vi "Read from Config File-Rev4.vi"(4 "error in (no error)":errorcluster, 5 "Measurement Information In":T4={"Comments"="", "Directory Input"="", "Data file path"=path "C:/Data/EPR Data", "Scripting File"=path "C:/Data/Configuration Script.csv", "Save Data"=FALSE, "Tooth size (d11) [mm]"=0.0, "Tooth size (d12) [mm]"=0.0, "Tooth size (d21) [mm]"=0.0, "Tooth size (d22) [mm]"=0.0, "Dose of Tooth [Gy]"=0.0, "Safe Shutdown?"=FALSE, "Gases Available"=[], "Database Username"="", "Database Password"="", "Database Login URL"="", "Database Upload URL"="", "Database Success URL"="", "Database XML URL"="", "Database Resonator URL"="", "Session Number"=0, "Set #"=0, "Resonator Operator"="", "Session Type"="", "Tooth/Sample ID"="", "Volunteer ID"="", "Computer Operator"="", "Volunteer Type"="", "Site/Tooth Selection (T8,T9)"="", "Resonator"="", "Measurement Site"="", "Non-standard session?"=FALSE, "EPR DAQ Version"="", "Session Path"=path "C:/Data/EPR Data", "Chosen Applied State"="", "Chosen Initial State"="", "Time of Transition"="", "DAQ Mode"=enum."Engineering", "pO2/Scan [mmHg]"=[], "pO2/Set [mmHg]"=[], "Linewidth (HWHM)/Scan [Gauss]"=[], "Linewidth (HWHM)/Set [Gauss]"=[], "pO2 Conversion"="", "Dose Calibration Cluster"={"Dose Response"={"grand_mean"=0.0292016, "slope"=0.0188720543}, "Dose Correction"={"Sex"=1, "a0"=7.719669421, "a1"=-2.746550736, "a2"=-0.186490355, "a3"=0.041922063, "a4"=-0.849147359, "a5"=0.14330063, "a6"=0.019930219, "A_n"=40.0, "H_n"=10.12, "Dose Correction"=FALSE}, "Dose Reporting"={"Reporting is"=TRUE, "sd_threshold [AU]"=0.06, "sd_model [Gy]"=0.66, "dosimetric_threshold [Gy]"=2.0, "Add intrasession errors is"=FALSE, "Prior Radiation?"=FALSE}}, "OxyChip Slope"=0.0, "OxyChip Intercept"=0.0, "QA Mode"=enum."Select QA Mode", "QA Session?"=FALSE, "Sample Type"=enum."Empty Resonator", "Report pO2/Scan"=FALSE, "Skip End Session Save"=FALSE, "Number of sites"=enum."# Probes", "Recipient Name"="", "Sender Name"="", "Recipient Email"="", "Transition State History"=[], "pO2 Report Times"=[], "Temperature [C]"=0.0, "+Error pO2/Scan [mmHg]"=[], "-Error pO2/Scan [mmHg]"=[], "+Error pO2/Set [mmHg]"=[], "-Error pO2/Set [mmHg]"=[], "Oxy Phase Exclusion Tolerance [rad]"=0.0, "Oxy Center Exclusion Tolerance [%]"=0.0, "Oxy Exclude Unacceptable"=FALSE, "Oxy Unacceptable Estimate Flags"=[], "Save Session PPT"=FALSE, "Flagged Bad Sets"=[]} {"Oxy Center Exclusion Tolerance [%]" format="%#_9g"; "Oxy Phase Exclusion Tolerance [rad]" format="%#_9g"; "Temperature [C]" format="%#_9g"; "OxyChip Intercept" format="%#_9g"; "OxyChip Slope" format="%#_9g"; "Dose Calibration Cluster"."Dose Reporting"."dosimetric_threshold [Gy]" format="%#_9g"; "Dose Calibration Cluster"."Dose Reporting"."sd_model [Gy]" format="%#_9g"; "Dose Calibration Cluster"."Dose Reporting"."sd_threshold [AU]" format="%#_9g"; "Dose Calibration Cluster"."Dose Correction"."H_n" format="%#_9g"; "Dose Calibration Cluster"."Dose Correction"."A_n" format="%#_9g"; "Dose Calibration Cluster"."Dose Correction"."a6" format="%#.9g"; "Dose Calibration Cluster"."Dose Correction"."a5" format="%#.9g"; "Dose Calibration Cluster"."Dose Correction"."a4" format="%#.9g"; "Dose Calibration Cluster"."Dose Correction"."a3" format="%#.9g"; "Dose Calibration Cluster"."Dose Correction"."a2" format="%#.9g"; "Dose Calibration Cluster"."Dose Correction"."a1" format="%#.9g"; "Dose Calibration Cluster"."Dose Correction"."a0" format="%#.9g"; "Dose Calibration Cluster"."Dose Correction"."Sex" items=["Male"=1, "Female"=0]; "Dose Calibration Cluster"."Dose Response"."slope" format="%#_9g"; "Dose Calibration Cluster"."Dose Response"."grand_mean" format="%#_9g"}, 6 "Hardware Parameters In":T3={"Scan Calibration [G/V]"=0.0, "Modulation Calibration [G/V]"=0.0, "Modulation Phase [deg]"=0.0, "Modulation Frequency [Hz]"=0.0, "Attenuation [dB]"=0, "Input Channel Count"=0, "Time constant"=7, "Sensitivity"=17, "Frequency Output Voltage [V]"=0.0, "Phase Output Voltage [V]"=0.0, "Lock-in Offset Compensation"=FALSE, "RF [GHz]"=0.0, "Q Start"=0.0, "Q End"=0.0, "Balance"=0.0, "Phase Error"=0.0, "AFC Error"=0.0, "AFC"=FALSE, "Magnet Rotation"=FALSE, "Balance Scaling Factor"=1.0, "Phase Error Scaling Factor"=1.0, "AFC Error Scaling Factor"=1.0, "Frequency Counter ID"="", "Sweep Waveform"=enum."Sawtooth", "Q-Factor Scale"=0.0, " Q-Data Scale"=0.0, " Q-Data Offset"=0.0, "Magnet Rotation Slope"=0.0, "Magnet Rotation Offset"=0.0, "Phase Sweep Resolution"=0.0, "Hardware Version Number"="", "Spectrometer ID Number"=0, "Spectrometer Name"="", "Lock in Saturation"=0.0, "Balance Threshold"=0.0, "Phase Error Threshold"=0.0, "AFC Error Threshold"=0.0, "Linear Actuator Length"=0.0, "Lock-in OK?"=FALSE, "Ignore Lock-in Comm. Failure"=FALSE, "Gradient Addresses"=[], "Gradient Calibrations [G/A*mm]"=[], "Gradient Power Supplies"=[], "Lock-in Address"="", "Magnet Type"=enum."RRI", "Camera Names"=[], "Sweep Limit [Gauss]"=0.0, "Modulation Limit [Gauss]"=0.0, "Balance Threshold Exceeded?"=FALSE, "Phase Threshold Exceeded?"=FALSE, "AFC Threshold Exceeded?"=FALSE, "Consecutive Re-tune attempts"=0, "Reverse Sweep Slope [sec]"=0.0, "Reverse Sweep Offset [G]"=0.0, "AFC Field Correction [V/MHz]"=0.0, "Active Gradients (X Y Z)"=[], "SpO2 Calibration [SpO2/V]"=1.0, "Heart Rate Calibration [BPM/V]"=1.0, "Thermocouple Channel"=""} {"Sensitivity" items=["", "2 nV", "5 nV", "10 nV", "20 nV", "50 nV", "100 nV", "200 nV", "500 nV", "1 uV", "2 uV", "5 uV", "10 uV", "20 uV", "50 uV", "100 uV", "200 uV", "500 uV", "1 mV", "2 mV", "5 mV", "10 mV", "20 mV", "50 mV", "100 mV", "200 mV", "500 mV", "1 V"]; "Time constant" items=["10 us", "20 us", "40 us", "80 us", "160 us", "320 us", "640 us", "5 ms", "10 ms", "20 ms", "50 ms", "100 ms", "200 ms", "500 ms", "1 s", "2 s", "5 s", "10 s", "20 s", "50 s", "100 s", "200 s", "500 s", "1 ks", "2 ks", "5 ks", "10 ks", "20 ks", "50 ks", "100 ks"]}, 7 "Acquisition Parameters In":T2={"Magnet Angle [deg]"=0.0, "Magnet Angles [deg]"=[], "DeltaVpp [v]"=0.0, "SEM [v]"=0.0, "DeltaVpp Thresh [v]"=0.0, "SEM Thresh [v]"=0.0, "Adaptive Processing"=FALSE, "Acquire Q"=FALSE, "Acquire Photos"=FALSE, "Adaptive Tuning"=FALSE, "Automated Matching"=FALSE, "X-Gradient [G/mm]"=0.0, "Y-Gradient [G/mm]"=0.0, "Z-Gradient [G/mm]"=0.0, "Central Field [G]"=0.0, "Scan Width [G]"=0.0, "Mod. Amp. [G]"=0.0, "Scan Time [s]"=0.0, "Pre-Scan Delay [ms]"=0, "Measurement Timeout [s]"=0.0, "Electromagnet Main Field [G]"=0.0, "Locked Central Field [G]"=0.0, "Scans Excluded"=0, "Scans Completed"=0, "No. Scans/Set"=0, "No. Scans for SNR"=0, "Field Locked Frequency [GHz]"=0.0, "Auto Set-based Field Center"=FALSE, "Prompt for oxy acquisition updates"=FALSE, "Oxy QA Scan?"=FALSE, "Exclude Bad Data"=FALSE, "Optimizing RF Power"=FALSE, "Gradients on/off"=FALSE, "Running Script"=TRUE, "Opto-Coupler Current [A]"=0.0, "Continuous Sweeping"=FALSE, "Sweep Rise Time [sec]"=0, "Reverse Sweep Central Field [G]"=0.0, "Forward Sweep Central Field [G]"=0.0, "Sweep Calibrated"=FALSE, "Modulation Calibrated"=FALSE, "First CheckCal Scan?"=FALSE, "AFC Field Correction"=FALSE, "OxyQAInit Scan Width [G]"=0.0, "OxyQAInit Mod. Amp. [G]"=0.0, "Scans Completed/Session"=0, "Acquire SpO2"=FALSE, "Acquire Temperature"=FALSE, "Over Mod"=FALSE} {"OxyQAInit Mod. Amp. [G]" min=0.0; "OxyQAInit Scan Width [G]" min=0.0; "Mod. Amp. [G]" min=0.0; "Scan Width [G]" min=0.0; "Central Field [G]" min=0.0; "Measurement Timeout [s]" min=0.0; "Scan Time [s]" min=0.0; "Z-Gradient [G/mm]" min=0.0; "SEM Thresh [v]" min=0.0; "SEM [v]" min=0.0; "DeltaVpp [v]" min=0.0}) -> (0 "error out":errorcluster, 1 "Measurement Information Out":T4={"Comments"="", "Directory Input"="", "Data file path"=path "C:/Data/EPR Data", "Scripting File"=path "C:/Data/Configuration Script.csv", "Save Data"=FALSE, "Tooth size (d11) [mm]"=0.0, "Tooth size (d12) [mm]"=0.0, "Tooth size (d21) [mm]"=0.0, "Tooth size (d22) [mm]"=0.0, "Dose of Tooth [Gy]"=0.0, "Safe Shutdown?"=FALSE, "Gases Available"=[], "Database Username"="", "Database Password"="", "Database Login URL"="", "Database Upload URL"="", "Database Success URL"="", "Database XML URL"="", "Database Resonator URL"="", "Session Number"=0, "Set #"=0, "Resonator Operator"="", "Session Type"="", "Tooth/Sample ID"="", "Volunteer ID"="", "Computer Operator"="", "Volunteer Type"="", "Site/Tooth Selection (T8,T9)"="", "Resonator"="", "Measurement Site"="", "Non-standard session?"=FALSE, "EPR DAQ Version"="", "Session Path"=path "C:/Data/EPR Data", "Chosen Applied State"="", "Chosen Initial State"="", "Time of Transition"="", "DAQ Mode"=enum."Engineering", "pO2/Scan [mmHg]"=[], "pO2/Set [mmHg]"=[], "Linewidth (HWHM)/Scan [Gauss]"=[], "Linewidth (HWHM)/Set [Gauss]"=[], "pO2 Conversion"="", "Dose Calibration Cluster"={"Dose Response"={"grand_mean"=0.0292016, "slope"=0.0188720543}, "Dose Correction"={"Sex"=1, "a0"=7.719669421, "a1"=-2.746550736, "a2"=-0.186490355, "a3"=0.041922063, "a4"=-0.849147359, "a5"=0.14330063, "a6"=0.019930219, "A_n"=40.0, "H_n"=10.12, "Dose Correction"=FALSE}, "Dose Reporting"={"Reporting is"=TRUE, "sd_threshold [AU]"=0.06, "sd_model [Gy]"=0.66, "dosimetric_threshold [Gy]"=2.0, "Add intrasession errors is"=FALSE, "Prior Radiation?"=FALSE}}, "OxyChip Slope"=0.0, "OxyChip Intercept"=0.0, "QA Mode"=enum."Select QA Mode", "QA Session?"=FALSE, "Sample Type"=enum."Empty Resonator", "Report pO2/Scan"=FALSE, "Skip End Session Save"=FALSE, "Number of sites"=enum."# Probes", "Recipient Name"="", "Sender Name"="", "Recipient Email"="", "Transition State History"=[], "pO2 Report Times"=[], "Temperature [C]"=0.0, "+Error pO2/Scan [mmHg]"=[], "-Error pO2/Scan [mmHg]"=[], "+Error pO2/Set [mmHg]"=[], "-Error pO2/Set [mmHg]"=[], "Oxy Phase Exclusion Tolerance [rad]"=0.0, "Oxy Center Exclusion Tolerance [%]"=0.0, "Oxy Exclude Unacceptable"=FALSE, "Oxy Unacceptable Estimate Flags"=[], "Save Session PPT"=FALSE, "Flagged Bad Sets"=[]} {"Oxy Center Exclusion Tolerance [%]" format="%#_9g"; "Oxy Phase Exclusion Tolerance [rad]" format="%#_9g"; "Temperature [C]" format="%#_9g"; "OxyChip Intercept" format="%#_9g"; "OxyChip Slope" format="%#_9g"; "Dose Calibration Cluster"."Dose Reporting"."dosimetric_threshold [Gy]" format="%#_9g"; "Dose Calibration Cluster"."Dose Reporting"."sd_model [Gy]" format="%#_9g"; "Dose Calibration Cluster"."Dose Reporting"."sd_threshold [AU]" format="%#_9g"; "Dose Calibration Cluster"."Dose Correction"."H_n" format="%#_9g"; "Dose Calibration Cluster"."Dose Correction"."A_n" format="%#_9g"; "Dose Calibration Cluster"."Dose Correction"."a6" format="%#.9g"; "Dose Calibration Cluster"."Dose Correction"."a5" format="%#.9g"; "Dose Calibration Cluster"."Dose Correction"."a4" format="%#.9g"; "Dose Calibration Cluster"."Dose Correction"."a3" format="%#.9g"; "Dose Calibration Cluster"."Dose Correction"."a2" format="%#.9g"; "Dose Calibration Cluster"."Dose Correction"."a1" format="%#.9g"; "Dose Calibration Cluster"."Dose Correction"."a0" format="%#.9g"; "Dose Calibration Cluster"."Dose Correction"."Sex" items=["Male"=1, "Female"=0]; "Dose Calibration Cluster"."Dose Response"."slope" format="%#_9g"; "Dose Calibration Cluster"."Dose Response"."grand_mean" format="%#_9g"}, 2 "Hardware Parameters Out":T3={"Scan Calibration [G/V]"=0.0, "Modulation Calibration [G/V]"=0.0, "Modulation Phase [deg]"=0.0, "Modulation Frequency [Hz]"=0.0, "Attenuation [dB]"=0, "Input Channel Count"=0, "Time constant"=7, "Sensitivity"=17, "Frequency Output Voltage [V]"=0.0, "Phase Output Voltage [V]"=0.0, "Lock-in Offset Compensation"=FALSE, "RF [GHz]"=0.0, "Q Start"=0.0, "Q End"=0.0, "Balance"=0.0, "Phase Error"=0.0, "AFC Error"=0.0, "AFC"=FALSE, "Magnet Rotation"=FALSE, "Balance Scaling Factor"=1.0, "Phase Error Scaling Factor"=1.0, "AFC Error Scaling Factor"=1.0, "Frequency Counter ID"="", "Sweep Waveform"=enum."Sawtooth", "Q-Factor Scale"=0.0, " Q-Data Scale"=0.0, " Q-Data Offset"=0.0, "Magnet Rotation Slope"=0.0, "Magnet Rotation Offset"=0.0, "Phase Sweep Resolution"=0.0, "Hardware Version Number"="", "Spectrometer ID Number"=0, "Spectrometer Name"="", "Lock in Saturation"=0.0, "Balance Threshold"=0.0, "Phase Error Threshold"=0.0, "AFC Error Threshold"=0.0, "Linear Actuator Length"=0.0, "Lock-in OK?"=FALSE, "Ignore Lock-in Comm. Failure"=FALSE, "Gradient Addresses"=[], "Gradient Calibrations [G/A*mm]"=[], "Gradient Power Supplies"=[], "Lock-in Address"="", "Magnet Type"=enum."RRI", "Camera Names"=[], "Sweep Limit [Gauss]"=0.0, "Modulation Limit [Gauss]"=0.0, "Balance Threshold Exceeded?"=FALSE, "Phase Threshold Exceeded?"=FALSE, "AFC Threshold Exceeded?"=FALSE, "Consecutive Re-tune attempts"=0, "Reverse Sweep Slope [sec]"=0.0, "Reverse Sweep Offset [G]"=0.0, "AFC Field Correction [V/MHz]"=0.0, "Active Gradients (X Y Z)"=[], "SpO2 Calibration [SpO2/V]"=1.0, "Heart Rate Calibration [BPM/V]"=1.0, "Thermocouple Channel"=""} {"Sensitivity" items=["", "2 nV", "5 nV", "10 nV", "20 nV", "50 nV", "100 nV", "200 nV", "500 nV", "1 uV", "2 uV", "5 uV", "10 uV", "20 uV", "50 uV", "100 uV", "200 uV", "500 uV", "1 mV", "2 mV", "5 mV", "10 mV", "20 mV", "50 mV", "100 mV", "200 mV", "500 mV", "1 V"]; "Time constant" items=["10 us", "20 us", "40 us", "80 us", "160 us", "320 us", "640 us", "5 ms", "10 ms", "20 ms", "50 ms", "100 ms", "200 ms", "500 ms", "1 s", "2 s", "5 s", "10 s", "20 s", "50 s", "100 s", "200 s", "500 s", "1 ks", "2 ks", "5 ks", "10 ks", "20 ks", "50 ks", "100 ks"]}, 3 "Acquisition Parameters Out":T2={"Magnet Angle [deg]"=0.0, "Magnet Angles [deg]"=[], "DeltaVpp [v]"=0.0, "SEM [v]"=0.0, "DeltaVpp Thresh [v]"=0.0, "SEM Thresh [v]"=0.0, "Adaptive Processing"=FALSE, "Acquire Q"=FALSE, "Acquire Photos"=FALSE, "Adaptive Tuning"=FALSE, "Automated Matching"=FALSE, "X-Gradient [G/mm]"=0.0, "Y-Gradient [G/mm]"=0.0, "Z-Gradient [G/mm]"=0.0, "Central Field [G]"=0.0, "Scan Width [G]"=0.0, "Mod. Amp. [G]"=0.0, "Scan Time [s]"=0.0, "Pre-Scan Delay [ms]"=0, "Measurement Timeout [s]"=0.0, "Electromagnet Main Field [G]"=0.0, "Locked Central Field [G]"=0.0, "Scans Excluded"=0, "Scans Completed"=0, "No. Scans/Set"=0, "No. Scans for SNR"=0, "Field Locked Frequency [GHz]"=0.0, "Auto Set-based Field Center"=FALSE, "Prompt for oxy acquisition updates"=FALSE, "Oxy QA Scan?"=FALSE, "Exclude Bad Data"=FALSE, "Optimizing RF Power"=FALSE, "Gradients on/off"=FALSE, "Running Script"=TRUE, "Opto-Coupler Current [A]"=0.0, "Continuous Sweeping"=FALSE, "Sweep Rise Time [sec]"=0, "Reverse Sweep Central Field [G]"=0.0, "Forward Sweep Central Field [G]"=0.0, "Sweep Calibrated"=FALSE, "Modulation Calibrated"=FALSE, "First CheckCal Scan?"=FALSE, "AFC Field Correction"=FALSE, "OxyQAInit Scan Width [G]"=0.0, "OxyQAInit Mod. Amp. [G]"=0.0, "Scans Completed/Session"=0, "Acquire SpO2"=FALSE, "Acquire Temperature"=FALSE, "Over Mod"=FALSE} {"OxyQAInit Mod. Amp. [G]" min=0.0; "OxyQAInit Scan Width [G]" min=0.0; "Mod. Amp. [G]" min=0.0; "Scan Width [G]" min=0.0; "Central Field [G]" min=0.0; "Measurement Timeout [s]" min=0.0; "Scan Time [s]" min=0.0; "Z-Gradient [G/mm]" min=0.0; "SEM Thresh [v]" min=0.0; "SEM [v]" min=0.0; "DeltaVpp [v]" min=0.0})   [LabVIEW 2016]
uses:
  Types/Acquisition Parameters.ctl
  Types/Hardware Parameters.ctl
  Types/Measurement Information.ctl
  Analysis/Dose Calculation and Reporting/Dose Calculation Control.ctl
  Types/Sample Type.ctl
  DAQ Management/Get Key Double.vi
  DAQ Management/Get Key U32.vi
  DAQ Management/Get Key String.vi
  DAQ Management/Get Key Bool.vi
  DAQ Management/Get Key I32.vi
  DAQ Management/Get Key Path.vi
panel:
  in  "Dose Calibration Cluster":T1={"Dose Response"={"grand_mean"=0.0292016, "slope"=0.0188720543}, "Dose Correction"={"Sex"=1, "a0"=7.719669421, "a1"=-2.746550736, "a2"=-0.186490355, "a3"=0.041922063, "a4"=-0.849147359, "a5"=0.14330063, "a6"=0.019930219, "A_n"=40.0, "H_n"=10.12, "Dose Correction"=FALSE}, "Dose Reporting"={"Reporting is"=TRUE, "sd_threshold [AU]"=0.06, "sd_model [Gy]"=0.66, "dosimetric_threshold [Gy]"=2.0, "Add intrasession errors is"=FALSE, "Prior Radiation?"=FALSE}} {"Dose Reporting"."dosimetric_threshold [Gy]" format="%#_9g"; "Dose Reporting"."sd_model [Gy]" format="%#_9g"; "Dose Reporting"."sd_threshold [AU]" format="%#_9g"; "Dose Correction"."H_n" format="%#_9g"; "Dose Correction"."A_n" format="%#_9g"; "Dose Correction"."a6" format="%#.9g"; "Dose Correction"."a5" format="%#.9g"; "Dose Correction"."a4" format="%#.9g"; "Dose Correction"."a3" format="%#.9g"; "Dose Correction"."a2" format="%#.9g"; "Dose Correction"."a1" format="%#.9g"; "Dose Correction"."a0" format="%#.9g"; "Dose Correction"."Sex" items=["Male"=1, "Female"=0]; "Dose Response"."slope" format="%#_9g"; "Dose Response"."grand_mean" format="%#_9g"}
  # "Gradients"
  # "Field"
  # "Scans and Sets"
  # "Timing"
  # "Adaptive Dosimetric \nData Processing"
  # "Bridge I/O"
  # "Magnet Rotation"
  # "Field Calibration"
  # "Lock In Amplifier"
  # "Spectrometer Information"
  # "DAQ Settings"
  # "Gradient Coils and Field"
  # "X"
  # "Y"
  # "Z"
  # "Q-Measurements"
  # "Session Information"
  # "Oximetric Data and Information"
  # "Email"
  # "Tooth Information"
  # "Database"
  # "Session Information"
  # "Oximetric Data and Information"
  # "Email"
  # "Tooth Information"
  # "Database"
  # "Bridge I/O"
  # "Magnet Rotation"
  # "Field Calibration"
  # "Lock In Amplifier"
  # "Spectrometer Information"
  # "DAQ Settings"
  # "Gradient Coils and Field"
  # "X"
  # "Y"
  # "Z"
  # "Q-Measurements"
  # "Gradients"
  # "Field"
  # "Scans and Sets"
  # "Timing"
  # "Adaptive Dosimetric \nData Processing"
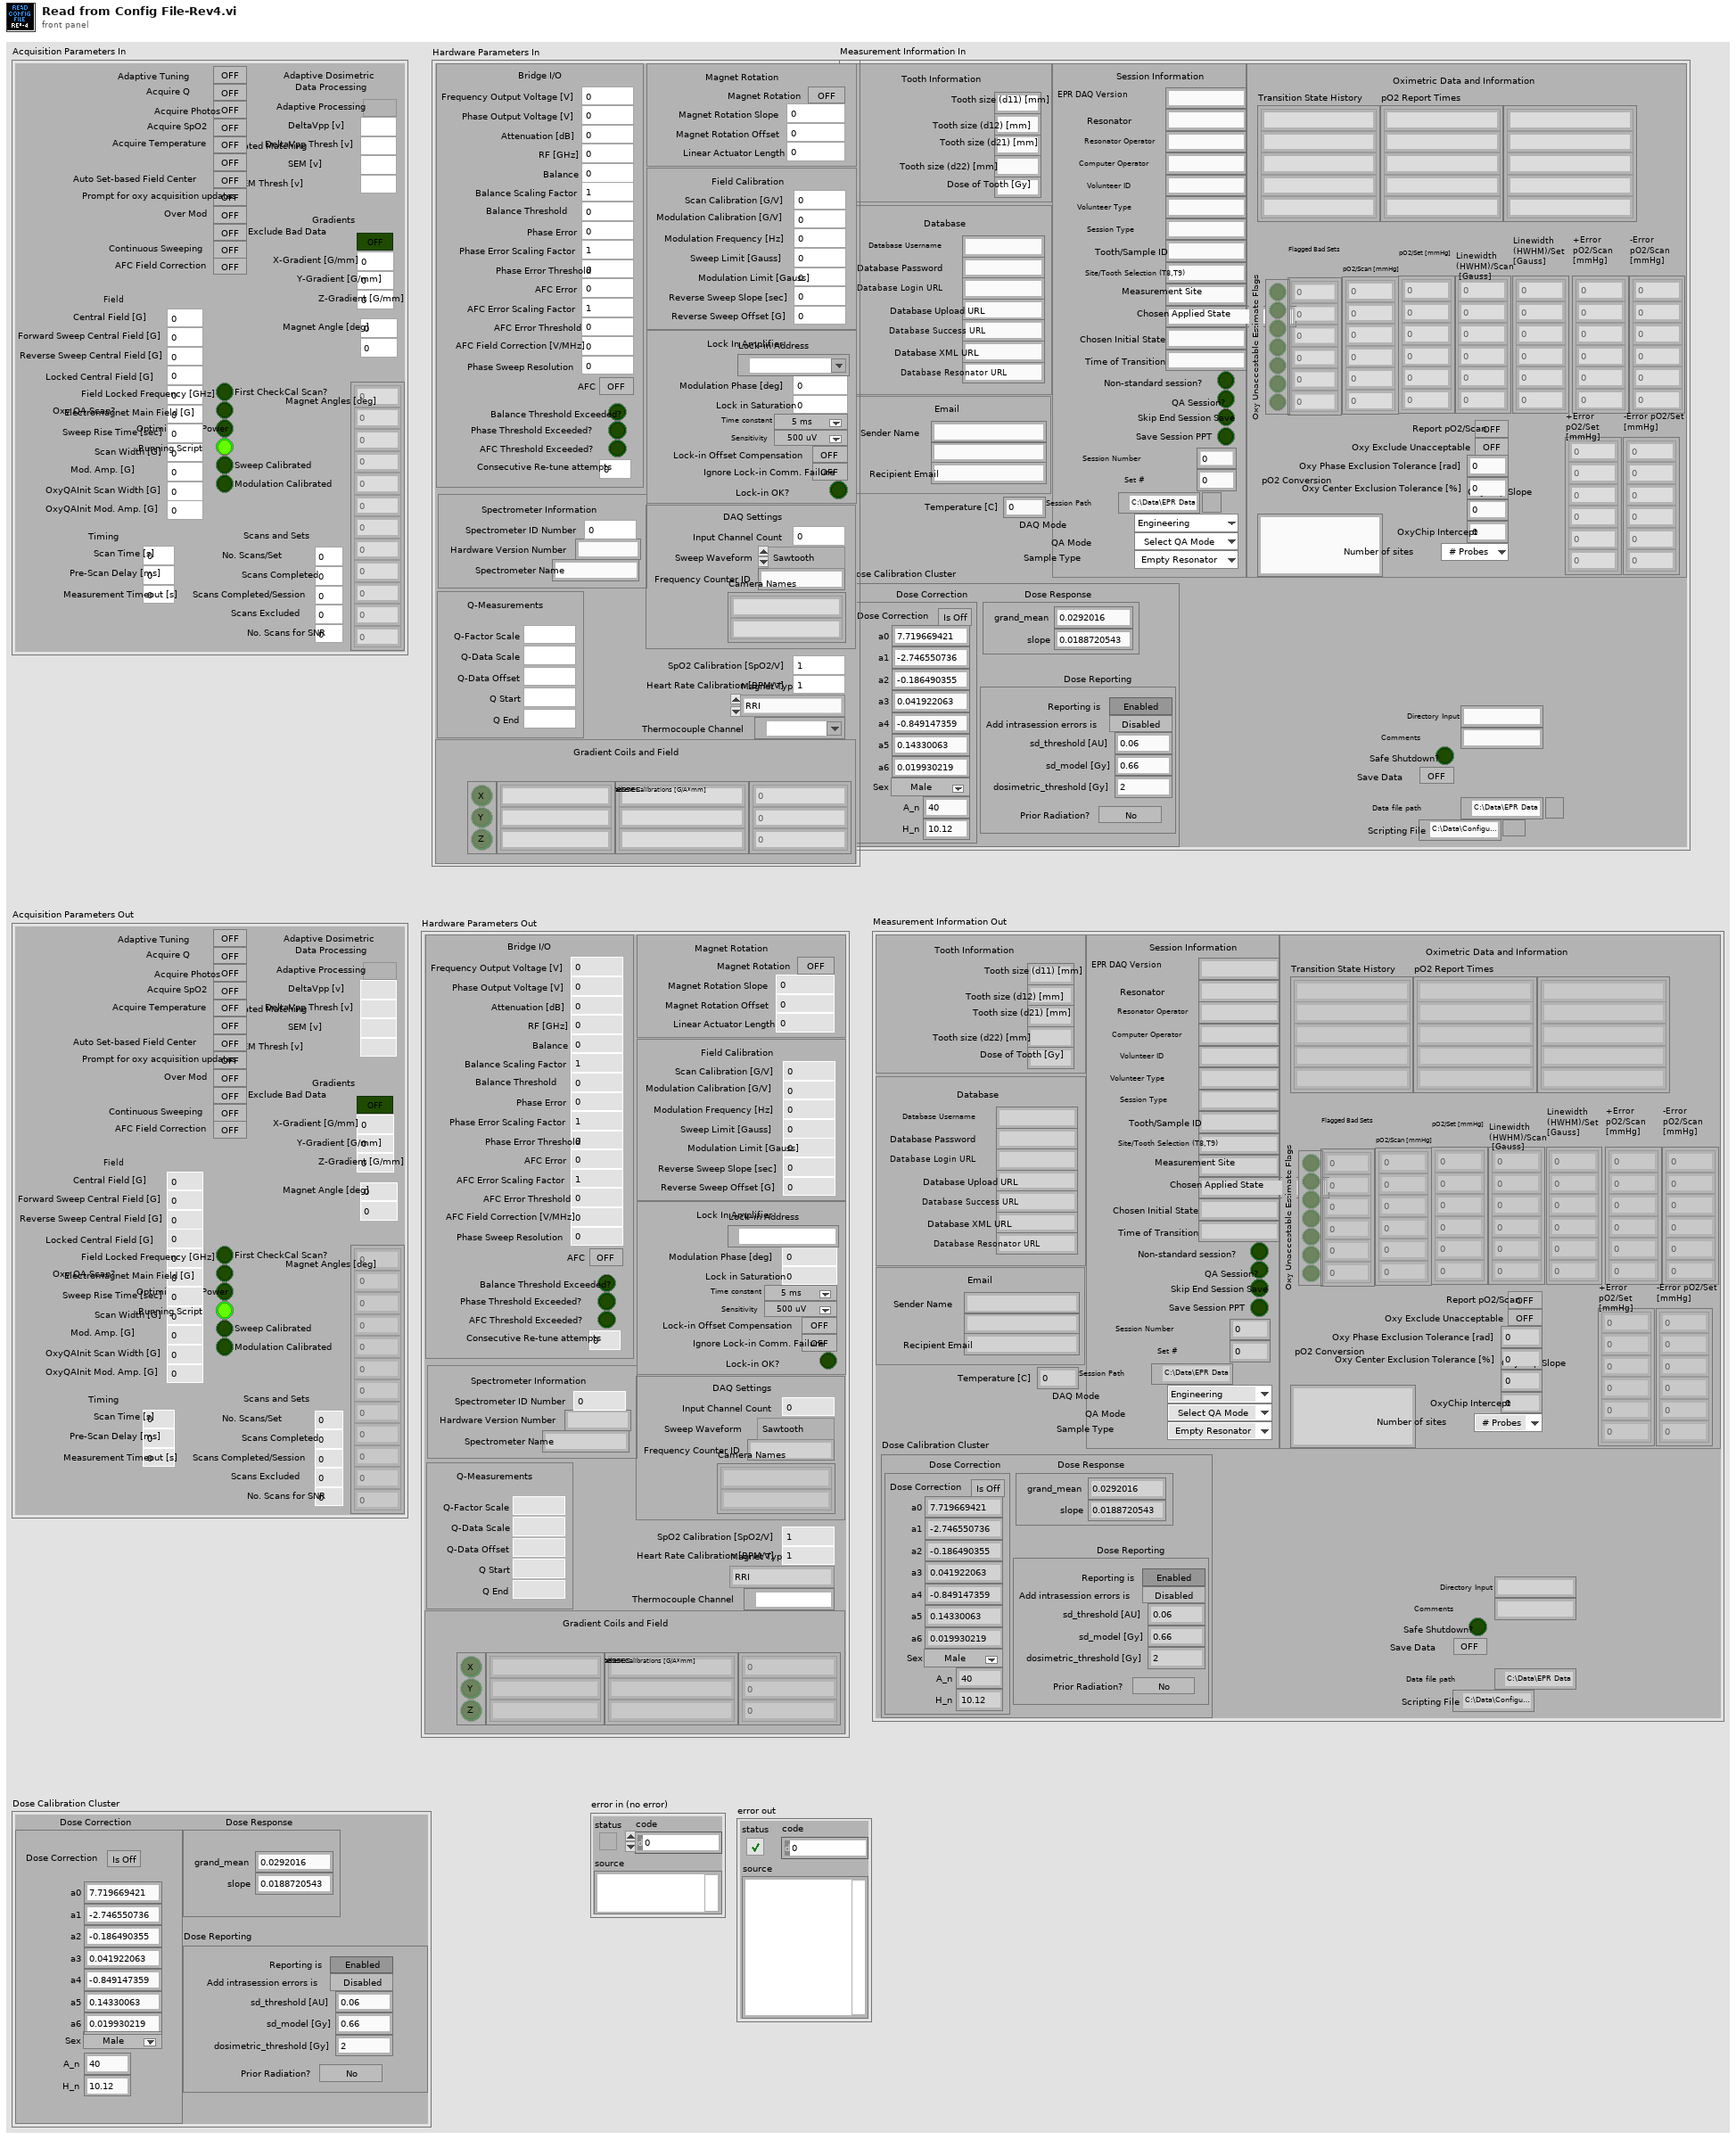
[diagram p1: front panel]
types:
  T1 = typedef "Dose Calculation Control.ctl" = cluster{"Dose Response":cluster{"grand_mean":dbl, "slope":dbl}, "Dose Correction":cluster{"Sex":u16, "a0":dbl, "a1":dbl, "a2":dbl, "a3":dbl, "a4":dbl, "a5":dbl, "a6":dbl, "A_n":dbl, "H_n":dbl, "Dose Correction":bool}, "Dose Reporting":cluster{"Reporting is":bool, "sd_threshold [AU]":dbl, "sd_model [Gy]":dbl, "dosimetric_threshold [Gy]":dbl, "Add intrasession errors is":bool, "Prior Radiation?":bool}}
  T2 = typedef "Acquisition Parameters.ctl" = cluster{"Magnet Angle [deg]":dbl, "Magnet Angles [deg]":dbl[], "DeltaVpp [v]":dbl, "SEM [v]":dbl, "DeltaVpp Thresh [v]":dbl, "SEM Thresh [v]":dbl, "Adaptive Processing":bool, "Acquire Q":bool, "Acquire Photos":bool, "Adaptive Tuning":bool, "Automated Matching":bool, "X-Gradient [G/mm]":dbl, "Y-Gradient [G/mm]":dbl, "Z-Gradient [G/mm]":dbl, "Central Field [G]":dbl, "Scan Width [G]":dbl, "Mod. Amp. [G]":dbl, "Scan Time [s]":dbl, "Pre-Scan Delay [ms]":u32, "Measurement Timeout [s]":dbl, "Electromagnet Main Field [G]":dbl, "Locked Central Field [G]":dbl, "Scans Excluded":u32, "Scans Completed":u32, "No. Scans/Set":u32, "No. Scans for SNR":u32, "Field Locked Frequency [GHz]":dbl, "Auto Set-based Field Center":bool, "Prompt for oxy acquisition updates":bool, "Oxy QA Scan?":bool, "Exclude Bad Data":bool, "Optimizing RF Power":bool, "Gradients on/off":bool, "Running Script":bool, "Opto-Coupler Current [A]":dbl, "Continuous Sweeping":bool, "Sweep Rise Time [sec]":u32, "Reverse Sweep Central Field [G]":dbl, "Forward Sweep Central Field [G]":dbl, "Sweep Calibrated":bool, "Modulation Calibrated":bool, "First CheckCal Scan?":bool, "AFC Field Correction":bool, "OxyQAInit Scan Width [G]":dbl, "OxyQAInit Mod. Amp. [G]":dbl, "Scans Completed/Session":u32, "Acquire SpO2":bool, "Acquire Temperature":bool, "Over Mod":bool}
  T3 = typedef "Hardware Parameters.ctl" = cluster{"Scan Calibration [G/V]":dbl, "Modulation Calibration [G/V]":dbl, "Modulation Phase [deg]":dbl, "Modulation Frequency [Hz]":dbl, "Attenuation [dB]":u16, "Input Channel Count":i32, "Time constant":u16, "Sensitivity":u16, "Frequency Output Voltage [V]":dbl, "Phase Output Voltage [V]":dbl, "Lock-in Offset Compensation":bool, "RF [GHz]":dbl, "Q Start":dbl, "Q End":dbl, "Balance":dbl, "Phase Error":dbl, "AFC Error":dbl, "AFC":bool, "Magnet Rotation":bool, "Balance Scaling Factor":dbl, "Phase Error Scaling Factor":dbl, "AFC Error Scaling Factor":dbl, "Frequency Counter ID":string, "Sweep Waveform":enum16{"Sine Wave", "Square Wave", "Sawtooth", "Triangle Wave"}, "Q-Factor Scale":dbl, " Q-Data Scale":dbl, " Q-Data Offset":dbl, "Magnet Rotation Slope":dbl, "Magnet Rotation Offset":dbl, "Phase Sweep Resolution":dbl, "Hardware Version Number":string, "Spectrometer ID Number":i32, "Spectrometer Name":string, "Lock in Saturation":dbl, "Balance Threshold":dbl, "Phase Error Threshold":dbl, "AFC Error Threshold":dbl, "Linear Actuator Length":dbl, "Lock-in OK?":bool, "Ignore Lock-in Comm. Failure":bool, "Gradient Addresses":string[], "Gradient Calibrations [G/A*mm]":dbl[], "Gradient Power Supplies":string[], "Lock-in Address":refnum<visa-resource-name>, "Magnet Type":enum16{"RRI", "BARDA", "Whole Body Permanent", "RRI Electromagnet"}, "Camera Names":string[], "Sweep Limit [Gauss]":dbl, "Modulation Limit [Gauss]":dbl, "Balance Threshold Exceeded?":bool, "Phase Threshold Exceeded?":bool, "AFC Threshold Exceeded?":bool, "Consecutive Re-tune attempts":i32, "Reverse Sweep Slope [sec]":dbl, "Reverse Sweep Offset [G]":dbl, "AFC Field Correction [V/MHz]":dbl, "Active Gradients (X Y Z)":bool[], "SpO2 Calibration [SpO2/V]":dbl, "Heart Rate Calibration [BPM/V]":dbl, "Thermocouple Channel":tag}
  T4 = typedef "Measurement Information.ctl" = cluster{"Comments":string, "Directory Input":string, "Data file path":path, "Scripting File":path, "Save Data":bool, "Tooth size (d11) [mm]":dbl, "Tooth size (d12) [mm]":dbl, "Tooth size (d21) [mm]":dbl, "Tooth size (d22) [mm]":dbl, "Dose of Tooth [Gy]":dbl, "Safe Shutdown?":bool, "Gases Available":string[], "Database Username":string, "Database Password":string, "Database Login URL":string, "Database Upload URL":string, "Database Success URL":string, "Database XML URL":string, "Database Resonator URL":string, "Session Number":i32, "Set #":u32, "Resonator Operator":string, "Session Type":string, "Tooth/Sample ID":string, "Volunteer ID":string, "Computer Operator":string, "Volunteer Type":string, "Site/Tooth Selection (T8,T9)":string, "Resonator":string, "Measurement Site":string, "Non-standard session?":bool, "EPR DAQ Version":string, "Session Path":path, "Chosen Applied State":string, "Chosen Initial State":string, "Time of Transition":string, "DAQ Mode":enum16{"Engineering", "Dosimetry", "Oximetry"}, "pO2/Scan [mmHg]":dbl[][], "pO2/Set [mmHg]":dbl[][], "Linewidth (HWHM)/Scan [Gauss]":dbl[][], "Linewidth (HWHM)/Set [Gauss]":dbl[][], "pO2 Conversion":string, "Dose Calibration Cluster":T1, "OxyChip Slope":dbl, "OxyChip Intercept":dbl, "QA Mode":enum16{"Select QA Mode", "QA-Start/End", "QA-Mid", "QA-Weekly", "QA-Eng", "Check Calibration"}, "QA Session?":bool, "Sample Type":T5, "Report pO2/Scan":bool, "Skip End Session Save":bool, "Number of sites":enum16{"# Probes", "1", "2", "3", "4"}, "Recipient Name":string, "Sender Name":string, "Recipient Email":string, "Transition State History":string[], "pO2 Report Times":string[], "Temperature [C]":dbl, "+Error pO2/Scan [mmHg]":dbl[][], "-Error pO2/Scan [mmHg]":dbl[][], "+Error pO2/Set [mmHg]":dbl[][], "-Error pO2/Set [mmHg]":dbl[][], "Oxy Phase Exclusion Tolerance [rad]":dbl, "Oxy Center Exclusion Tolerance [%]":dbl, "Oxy Exclude Unacceptable":bool, "Oxy Unacceptable Estimate Flags":bool[], "Save Session PPT":bool, "Flagged Bad Sets":u32[]}
  T5 = typedef "Sample Type.ctl" = enum16{"Empty Resonator", "IRS", "BallZero", "Irradiated Tooth", "Non-irradiated Tooth", "OxyChip", "LiPc", "PDT", "India Ink"}
  T6 = enum16{"RRI", "BARDA", "Whole Body Permanent", "RRI Electromagnet"}
  T7 = enum16{"Sine Wave", "Square Wave", "Sawtooth", "Triangle Wave"}
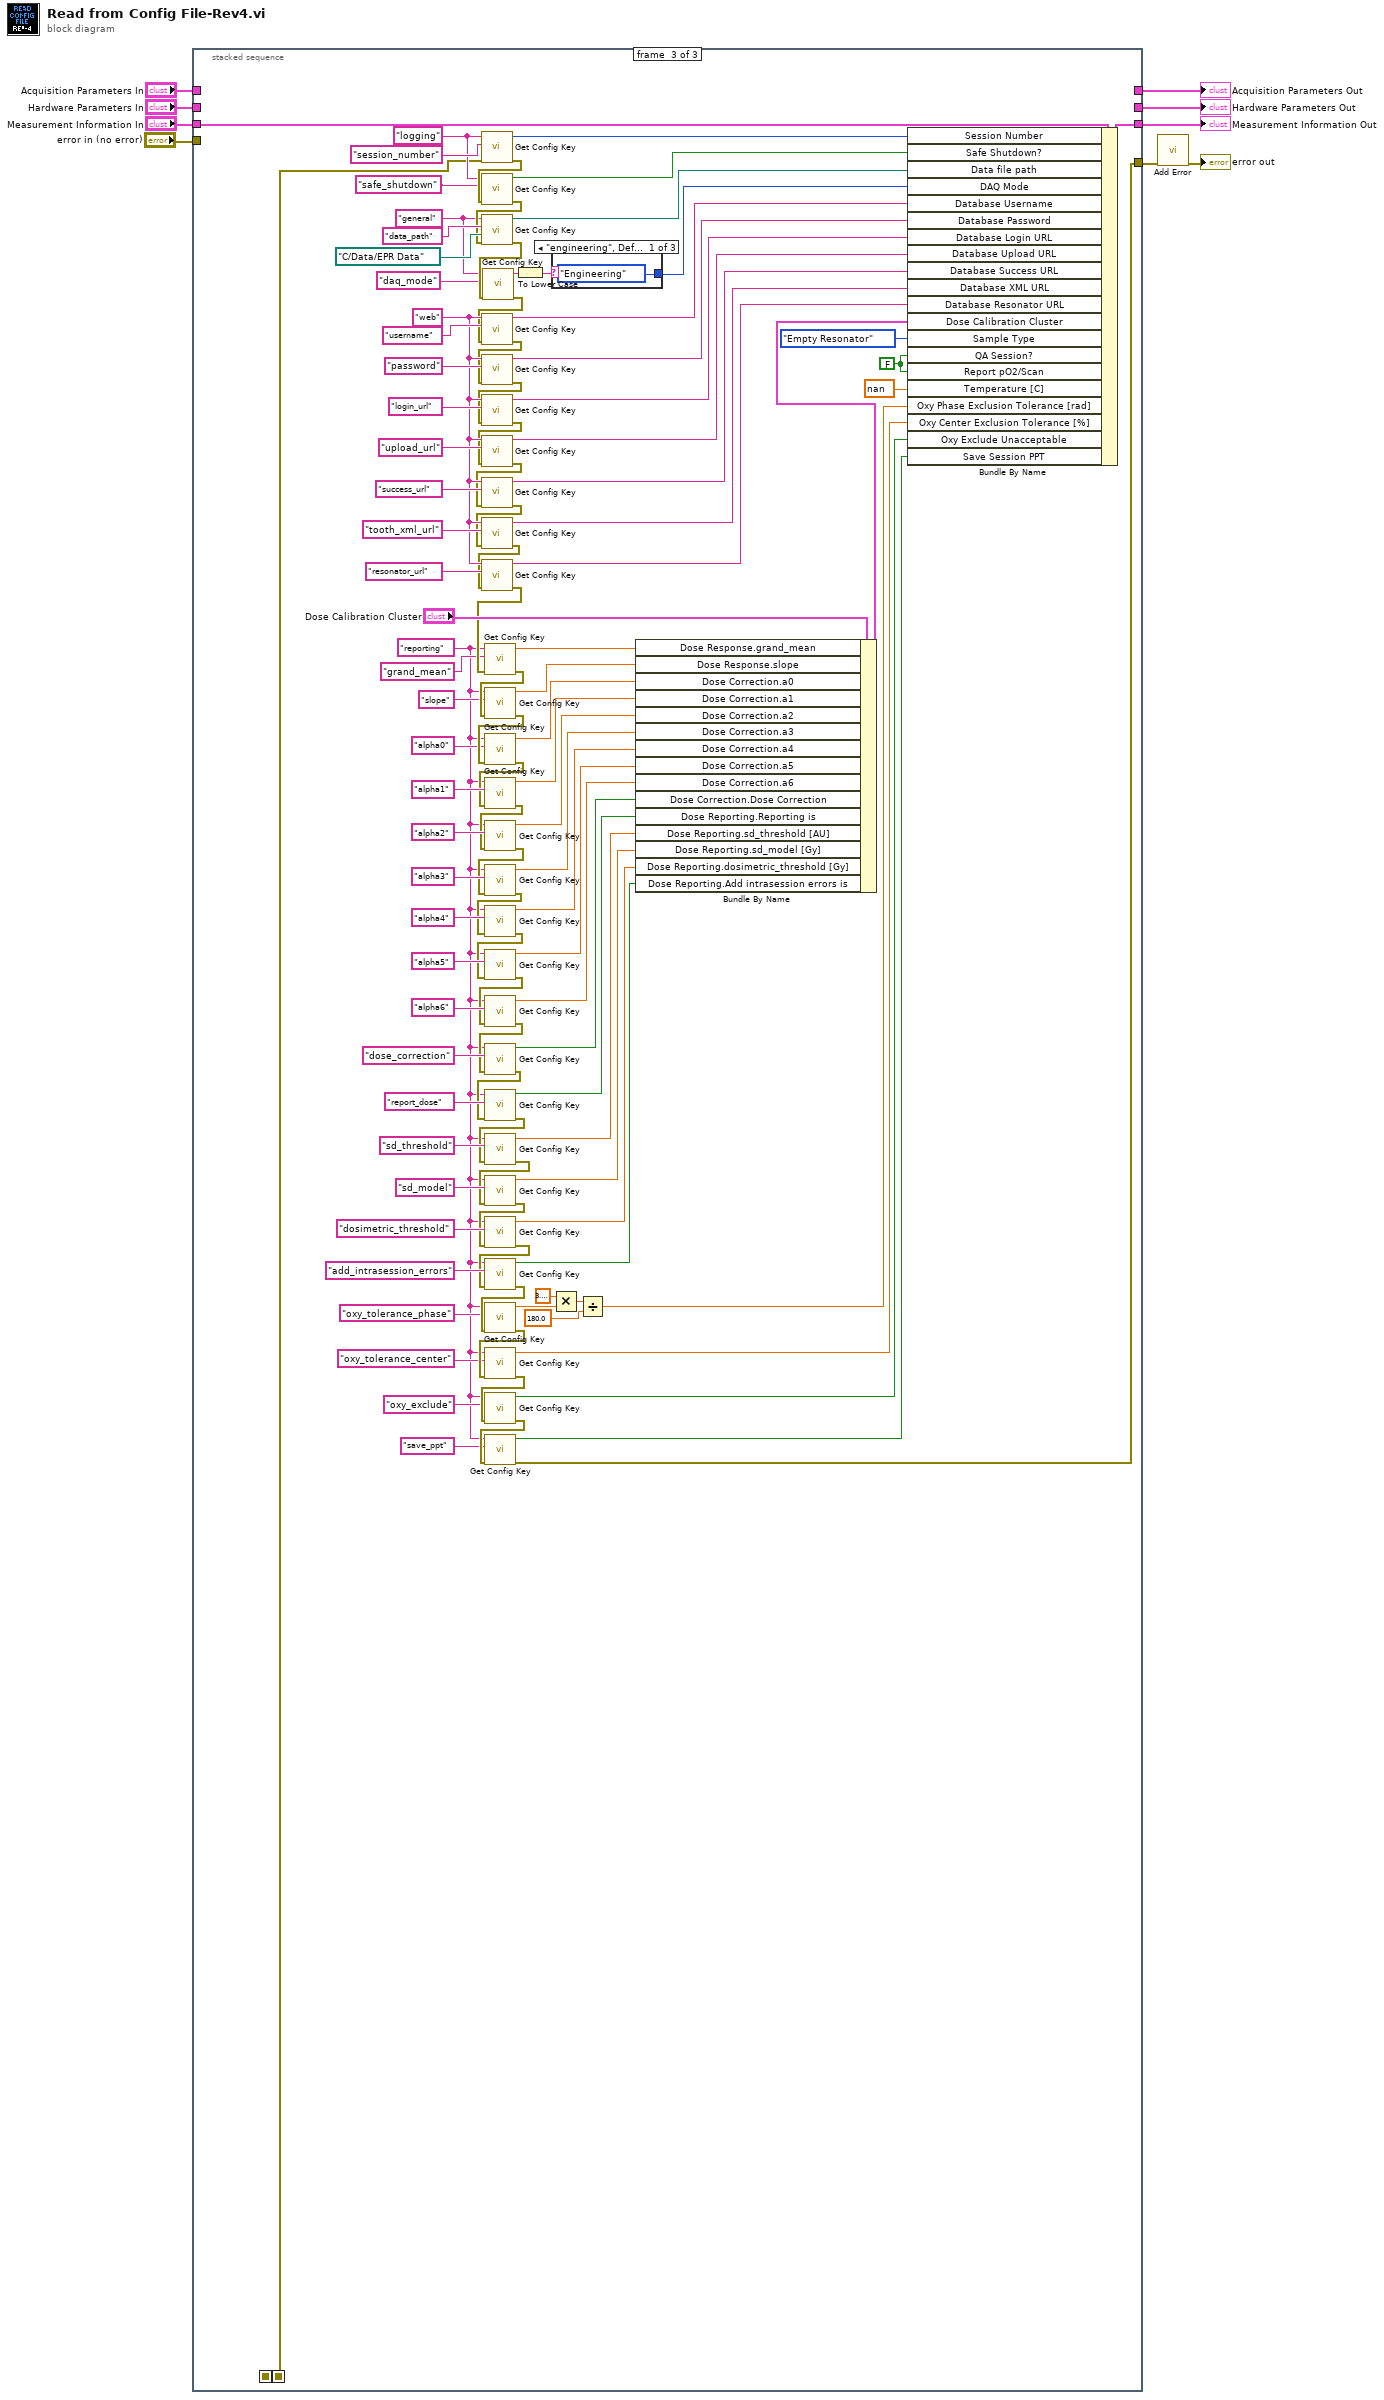
[diagram p0: block diagram]
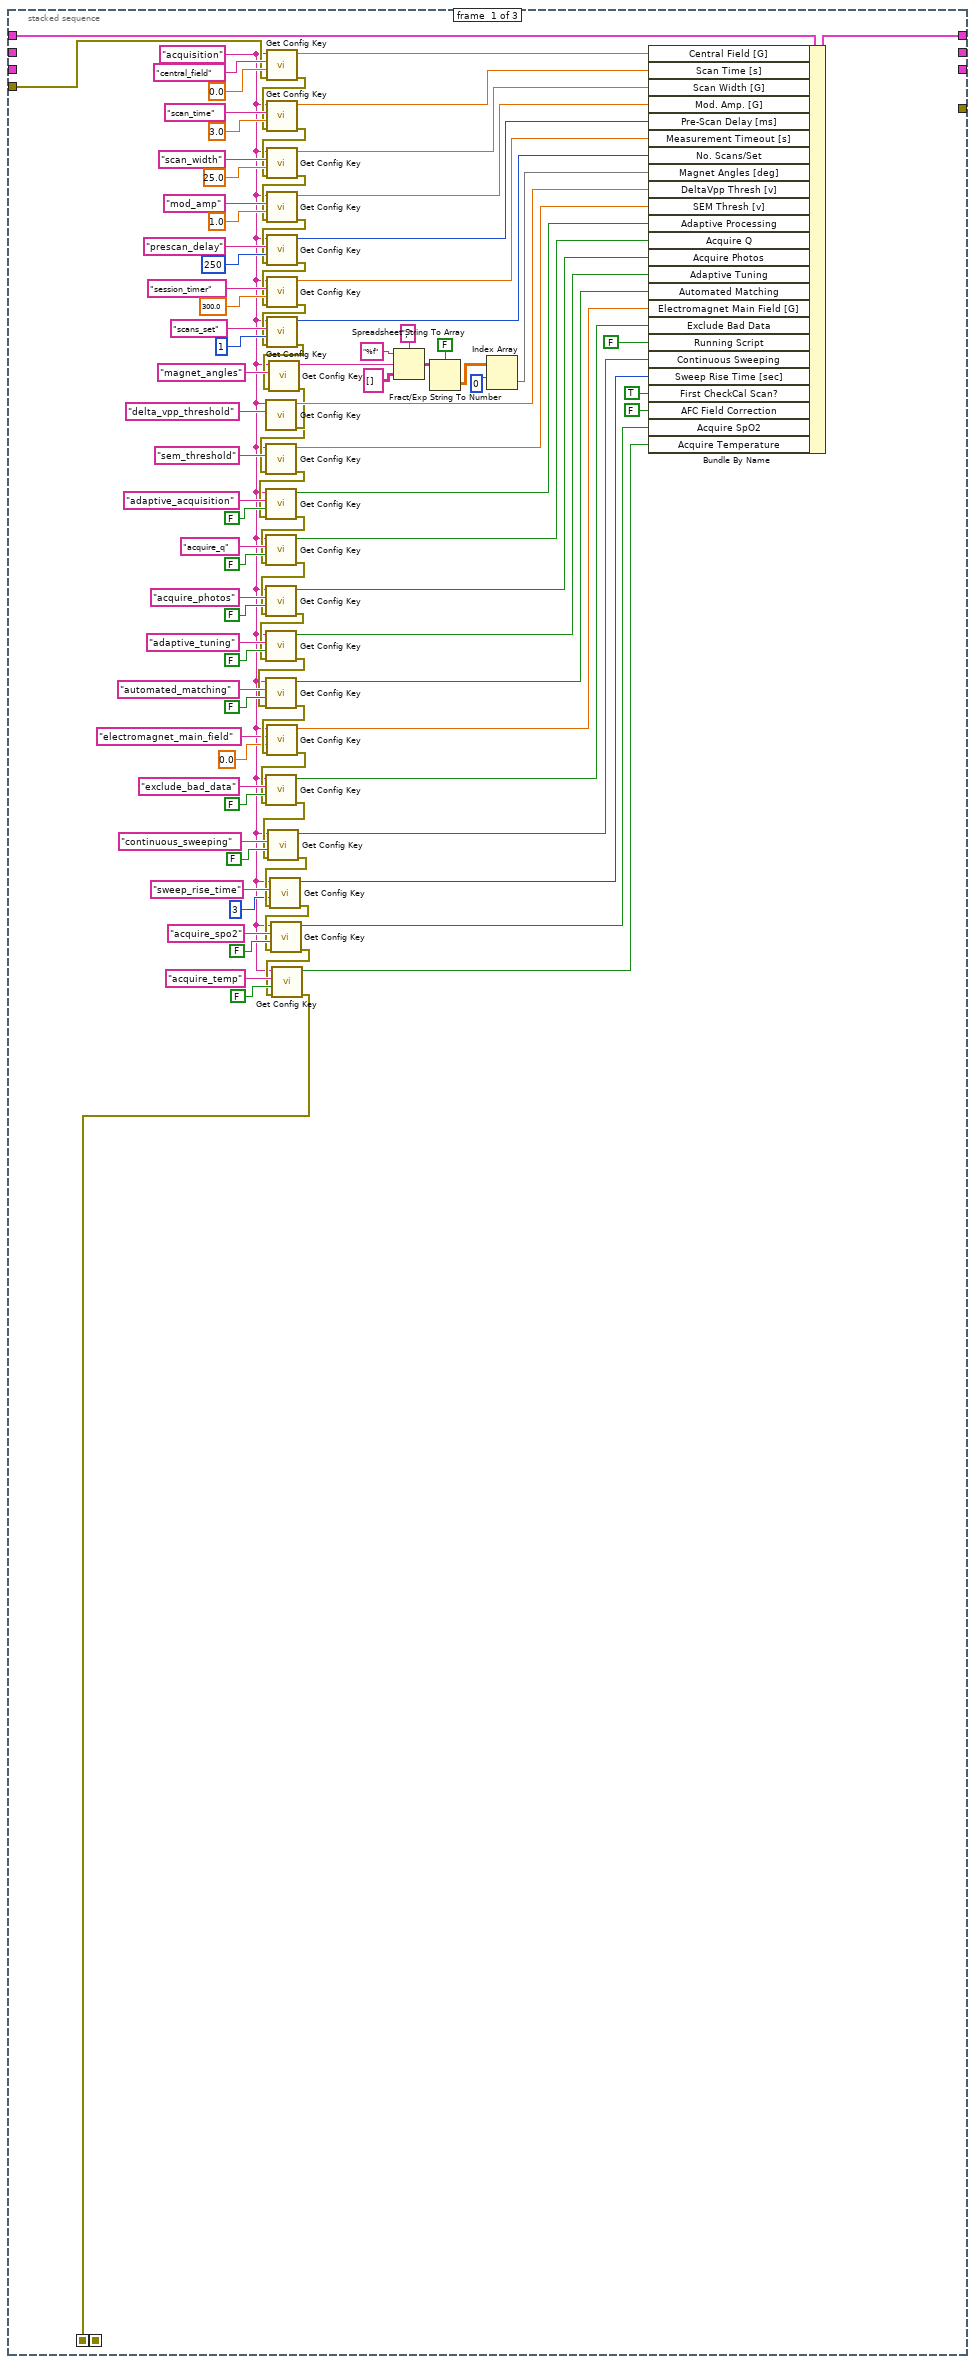
[diagram p2: hidden frame]
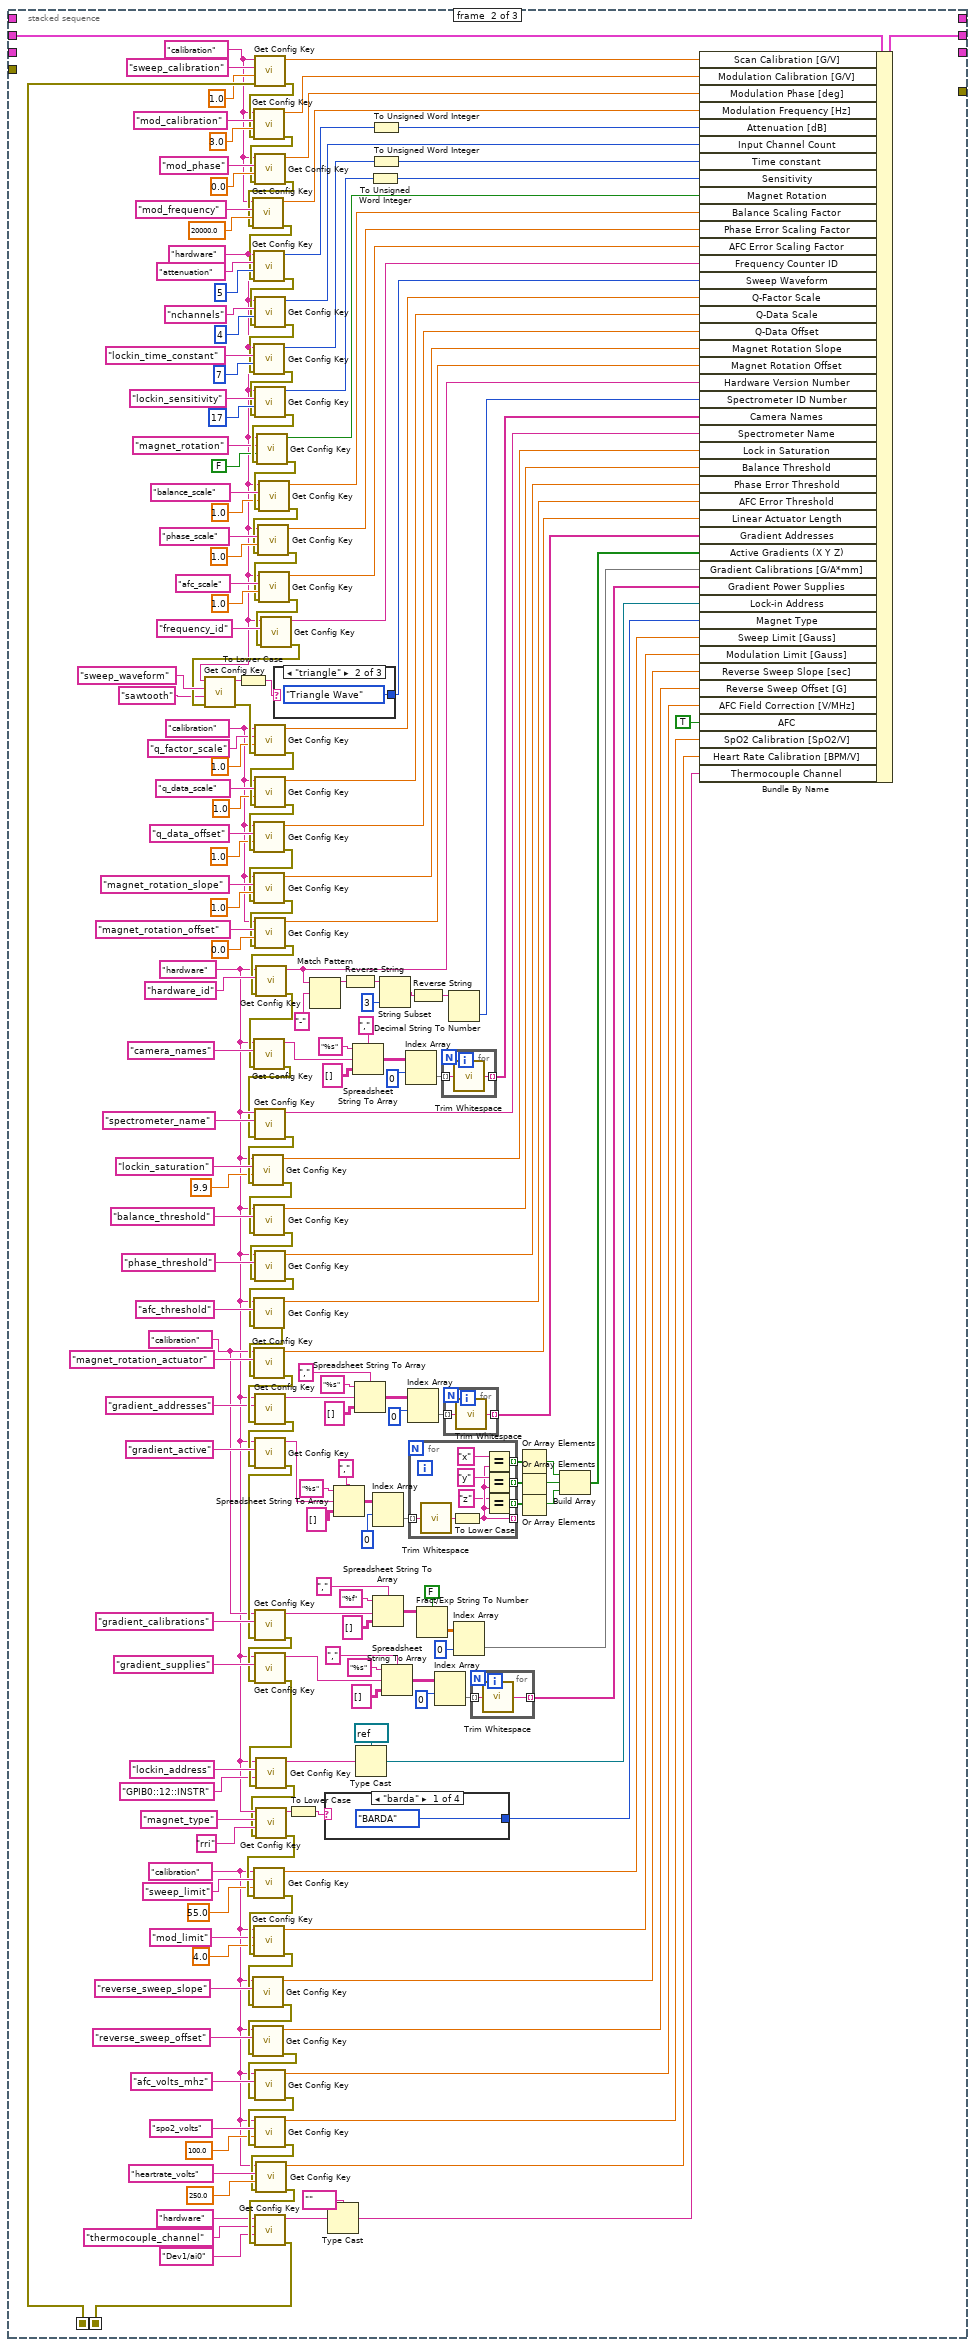
[diagram p3: hidden frame]
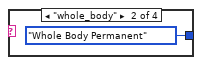
[diagram p4: hidden frame]
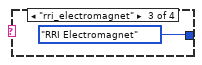
[diagram p5: hidden frame]
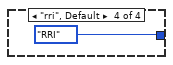
[diagram p6: hidden frame]
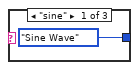
[diagram p7: hidden frame]
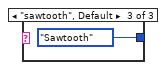
[diagram p8: hidden frame]
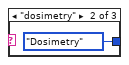
[diagram p9: hidden frame]
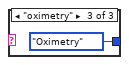
[diagram p10: hidden frame]
diagram:
  n1 = stacked-sequence {
    seq-local: [w11 _ _] -> [_ w322 _]
    seq-local: [_ w111 _] -> [_ _ w424]
    tunnel: "Measurement Information In" -> [_ _ w456]
    tunnel: [_ _ w437] -> w8
    tunnel: "Acquisition Parameters In" -> [w105 _ _]
    tunnel: "Hardware Parameters In" -> [_ w325 _]
    tunnel: [w104 _ _] -> w5
    tunnel: [_ w324 _] -> w4
    tunnel: [_ _ w352] -> w2
    tunnel: "error in (no error)" -> [w39 _ _]
    frame #0 {
      w12 = "acquisition" ("section")
      n2 = call-poly "Get Config Key.vi"("error in (no error)"=w39, "default value"=0.0, "key"="central_field", "section"=w12) -> ("error out"=w53:errorcluster, "value"=w102:dbl)  [unwired: 6 in]
      n3 = call-poly "Get Config Key.vi"("error in (no error)"=w53, "default value"=3.0, "key"="scan_time", "section"=w12) -> ("error out"=w52:errorcluster, "value"=w98:dbl)  [unwired: 6 in]
      n4 = call-poly "Get Config Key.vi"("error in (no error)"=w52, "default value"=25.0, "key"="scan_width", "section"=w12) -> ("error out"=w51:errorcluster, "value"=w95:dbl)  [unwired: 6 in]
      n5 = call-poly "Get Config Key.vi"("error in (no error)"=w51, "default value"=1.0, "key"="mod_amp", "section"=w12) -> ("error out"=w50:errorcluster, "value"=w92:dbl)  [unwired: 6 in]
      n6 = call-poly "Get Config Key.vi"("error in (no error)"=w50, "default value"=u32 250, "key"="prescan_delay", "section"=w12) -> ("error out"=w49:errorcluster, "value"=w89:u32)  [unwired: 6 in]
      n7 = call-poly "Get Config Key.vi"("error in (no error)"=w49, "default value"=300.0, "key"="session_timer", "section"=w12) -> ("error out"=w48:errorcluster, "value"=w86:dbl)  [unwired: 6 in]
      n8 = call-poly "Get Config Key.vi"("error in (no error)"=w48, "default value"=u32 1, "key"="scans_set", "section"=w12) -> ("error out"=w47:errorcluster, "value"=w83:u32)  [unwired: 6 in]
      n9 = call-poly "Get Config Key.vi"("error in (no error)"=w47, "key"="magnet_angles", "section"=w12) -> ("error out"=w46:errorcluster, "value"=w74:string)  [unwired: 7 in]
      n10 = call-poly "Get Config Key.vi"("error in (no error)"=w46, "key"="delta_vpp_threshold", "section"=w12) -> ("error out"=w45:errorcluster, "value"=w71:dbl)  [unwired: 7 in]
      n11 = call-poly "Get Config Key.vi"("error in (no error)"=w45, "key"="sem_threshold", "section"=w12) -> ("error out"=w44:errorcluster, "value"=w69:dbl)  [unwired: 7 in]
      n12 = call-poly "Get Config Key.vi"("error in (no error)"=w44, "default value"=FALSE, "key"="adaptive_acquisition", "section"=w12) -> ("error out"=w43:errorcluster, "value"=w66:bool)  [unwired: 6 in]
      n13 = call-poly "Get Config Key.vi"("error in (no error)"=w43, "default value"=FALSE, "key"="acquire_q", "section"=w12) -> ("error out"=w42:errorcluster, "value"=w63:bool)  [unwired: 6 in]
      n14 = call-poly "Get Config Key.vi"("error in (no error)"=w42, "default value"=FALSE, "key"="acquire_photos", "section"=w12) -> ("error out"=w41:errorcluster, "value"=w60:bool)  [unwired: 6 in]
      n15 = call-poly "Get Config Key.vi"("error in (no error)"=w41, "default value"=FALSE, "key"="adaptive_tuning", "section"=w12) -> ("error out"=w40:errorcluster, "value"=w57:bool)  [unwired: 6 in]
      n16 = call-poly "Get Config Key.vi"("error in (no error)"=w40, "default value"=FALSE, "key"="automated_matching", "section"=w12) -> ("error out"=w38:errorcluster, "value"=w54:bool)  [unwired: 6 in]
      n17 = call-poly "Get Config Key.vi"("error in (no error)"=w38, "default value"=0.0, "key"="electromagnet_main_field", "section"=w12) -> ("error out"=w32:errorcluster, "value"=w35:dbl)  [unwired: 6 in]
      n18 = call-poly "Get Config Key.vi"("error in (no error)"=w32, "default value"=FALSE, "key"="exclude_bad_data", "section"=w12) -> ("error out"=w27:errorcluster, "value"=w31:bool)  [unwired: 6 in]
      n19 = call-poly "Get Config Key.vi"("error in (no error)"=w27, "default value"=FALSE, "key"="continuous_sweeping", "section"=w12) -> ("error out"=w24:errorcluster, "value"=w26:bool)  [unwired: 6 in]
      n20 = call-poly "Get Config Key.vi"("error in (no error)"=w24, "default value"=u32 3, "key"="sweep_rise_time", "section"=w12) -> ("error out"=w17:errorcluster, "value"=w22:u32)  [unwired: 6 in]
      n21 = call-poly "Get Config Key.vi"("error in (no error)"=w17, "default value"=FALSE, "key"="acquire_spo2", "section"=w12) -> ("error out"=w13:errorcluster, "value"=w16:bool)  [unwired: 6 in]
      n22 = call-poly "Get Config Key.vi"("error in (no error)"=w13, "default value"=FALSE, "key"="acquire_temp", "section"=w12) -> ("error out"=w11:errorcluster, "value"=w10:bool)  [unwired: 6 in]
      n23 = Spreadsheet String To Array(delimiter (Tab)=",", format string="%f", spreadsheet string=w74, array type (2D Dbl)=string[][] []) -> (array=w78:string[][])
      n24 = Fract/Exp String To Number(use system decimal point (T)=FALSE, string=w78) -> (number=w80:dbl[][])  [unwired: 2 in, 1 out]
      n25 = Index Array(array=w80, index (row)=0) -> (element=w73:dbl[])  [unwired: 1 in]
      n26 = Bundle By Name(cluster=w105, "Central Field [G]"=w102, "Scan Time [s]"=w98, "Scan Width [G]"=w95, "Mod. Amp. [G]"=w92, "Pre-Scan Delay [ms]"=w89, "Measurement Timeout [s]"=w86, "No. Scans/Set"=w83, "Magnet Angles [deg]"=w73, "DeltaVpp Thresh [v]"=w71, "SEM Thresh [v]"=w69, "Adaptive Processing"=w66, "Acquire Q"=w63, "Acquire Photos"=w60, "Adaptive Tuning"=w57, "Automated Matching"=w54, "Electromagnet Main Field [G]"=w35, "Exclude Bad Data"=w31, "Running Script"=FALSE, "Continuous Sweeping"=w26, "Sweep Rise Time [sec]"=w22, "First CheckCal Scan?"=TRUE, "AFC Field Correction"=FALSE, "Acquire SpO2"=w16, "Acquire Temperature"=w10) -> (w104:T2)
    }
    frame #1 {
      w115 = "calibration" ("section")
      w189 = "calibration" ("section")
      w170 = "hardware" ("section")
      w240 = "calibration" ("section")
      w262 = "hardware" ("section")
      w305 = "calibration" ("section")
      n27 = call-poly "Get Config Key.vi"("error in (no error)"=w322, "default value"=1.0, "key"="sweep_calibration", "section"=w305) -> ("error out"=w317:errorcluster, "value"=w321:dbl)  [unwired: 6 in]
      n28 = call-poly "Get Config Key.vi"("error in (no error)"=w317, "default value"=3.0, "key"="mod_calibration", "section"=w305) -> ("error out"=w312:errorcluster, "value"=w316:dbl)  [unwired: 6 in]
      n29 = call-poly "Get Config Key.vi"("error in (no error)"=w312, "default value"=0.0, "key"="mod_phase", "section"=w305) -> ("error out"=w308:errorcluster, "value"=w313:dbl)  [unwired: 6 in]
      n30 = call-poly "Get Config Key.vi"("error in (no error)"=w308, "default value"=20000.0, "key"="mod_frequency", "section"=w305) -> ("error out"=w304:errorcluster, "value"=w309:dbl)  [unwired: 6 in]
      n31 = call-poly "Get Config Key.vi"("error in (no error)"=w304, "default value"=u32 5, "key"="attenuation", "section"=w262) -> ("error out"=w299:errorcluster, "value"=w302:u32)  [unwired: 6 in]
      n32 = call-poly "Get Config Key.vi"("error in (no error)"=w299, "default value"=4, "key"="nchannels", "section"=w262) -> ("error out"=w293:errorcluster, "value"=w298:i32)  [unwired: 6 in]
      n33 = call-poly "Get Config Key.vi"("error in (no error)"=w293, "default value"=u32 7, "key"="lockin_time_constant", "section"=w262) -> ("error out"=w290:errorcluster, "value"=w294:u32)  [unwired: 6 in]
      n34 = call-poly "Get Config Key.vi"("error in (no error)"=w290, "default value"=u32 17, "key"="lockin_sensitivity", "section"=w262) -> ("error out"=w287:errorcluster, "value"=w288:u32)  [unwired: 6 in]
      n35 = call-poly "Get Config Key.vi"("error in (no error)"=w287, "default value"=FALSE, "key"="magnet_rotation", "section"=w262) -> ("error out"=w282:errorcluster, "value"=w286:bool)  [unwired: 6 in]
      n36 = call-poly "Get Config Key.vi"("error in (no error)"=w282, "default value"=1.0, "key"="balance_scale", "section"=w262) -> ("error out"=w277:errorcluster, "value"=w280:dbl)  [unwired: 6 in]
      n37 = call-poly "Get Config Key.vi"("error in (no error)"=w277, "default value"=1.0, "key"="phase_scale", "section"=w262) -> ("error out"=w273:errorcluster, "value"=w276:dbl)  [unwired: 6 in]
      n38 = call-poly "Get Config Key.vi"("error in (no error)"=w273, "default value"=1.0, "key"="afc_scale", "section"=w262) -> ("error out"=w270:errorcluster, "value"=w272:dbl)  [unwired: 6 in]
      n39 = call-poly "Get Config Key.vi"("error in (no error)"=w270, "key"="frequency_id", "section"=w262) -> ("error out"=w267:errorcluster, "value"=w269:string)  [unwired: 7 in]
      n40 = call-poly "Get Config Key.vi"("error in (no error)"=w267, "default value"="sawtooth", "key"="sweep_waveform", "section"=w262) -> ("error out"=w261:errorcluster, "value"=w266:string)  [unwired: 6 in]
      n41 = To Lower Case(string=w266) -> (all lower case string=w265:string)
      n42 = call-poly "Get Config Key.vi"("error in (no error)"=w261, "default value"=1.0, "key"="q_factor_scale", "section"=w240) -> ("error out"=w257:errorcluster, "value"=w260:dbl)  [unwired: 6 in]
      n43 = call-poly "Get Config Key.vi"("error in (no error)"=w257, "default value"=1.0, "key"="q_data_scale", "section"=w240) -> ("error out"=w254:errorcluster, "value"=w256:dbl)  [unwired: 6 in]
      n44 = call-poly "Get Config Key.vi"("error in (no error)"=w254, "default value"=1.0, "key"="q_data_offset", "section"=w240) -> ("error out"=w247:errorcluster, "value"=w253:dbl)  [unwired: 6 in]
      n45 = call-poly "Get Config Key.vi"("error in (no error)"=w247, "default value"=1.0, "key"="magnet_rotation_slope", "section"=w240) -> ("error out"=w243:errorcluster, "value"=w246:dbl)  [unwired: 6 in]
      n46 = call-poly "Get Config Key.vi"("error in (no error)"=w243, "default value"=0.0, "key"="magnet_rotation_offset", "section"=w240) -> ("error out"=w239:errorcluster, "value"=w242:dbl)  [unwired: 6 in]
      n47 = call-poly "Get Config Key.vi"("error in (no error)"=w239, "key"="hardware_id", "section"=w170) -> ("error out"=w229:errorcluster, "value"=w233:string)  [unwired: 7 in]
      n48 = call-poly "Get Config Key.vi"("error in (no error)"=w229, "key"="camera_names", "section"=w170) -> ("error out"=w163:errorcluster, "value"=w156:string)  [unwired: 7 in]
      n49 = call-poly "Get Config Key.vi"("error in (no error)"=w163, "key"="spectrometer_name", "section"=w170) -> ("error out"=w225:errorcluster, "value"=w227:string)  [unwired: 7 in]
      n50 = call-poly "Get Config Key.vi"("error in (no error)"=w225, "default value"=9.9, "key"="lockin_saturation", "section"=w170) -> ("error out"=w221:errorcluster, "value"=w224:dbl)  [unwired: 6 in]
      n51 = call-poly "Get Config Key.vi"("error in (no error)"=w221, "key"="balance_threshold", "section"=w170) -> ("error out"=w218:errorcluster, "value"=w220:dbl)  [unwired: 7 in]
      n52 = call-poly "Get Config Key.vi"("error in (no error)"=w218, "key"="phase_threshold", "section"=w170) -> ("error out"=w215:errorcluster, "value"=w217:dbl)  [unwired: 7 in]
      n53 = call-poly "Get Config Key.vi"("error in (no error)"=w215, "key"="afc_threshold", "section"=w170) -> ("error out"=w212:errorcluster, "value"=w214:dbl)  [unwired: 7 in]
      n54 = call-poly "Get Config Key.vi"("error in (no error)"=w212, "key"="magnet_rotation_actuator", "section"=w189) -> ("error out"=w204:errorcluster, "value"=w211:dbl)  [unwired: 7 in]
      n55 = call-poly "Get Config Key.vi"("error in (no error)"=w204, "key"="gradient_addresses", "section"=w170) -> ("error out"=w199:errorcluster, "value"=w202:string)  [unwired: 7 in]
      n56 = call-poly "Get Config Key.vi"("error in (no error)"=w199, "key"="gradient_active", "section"=w170) -> ("error out"=w190:errorcluster, "value"=w125:string)  [unwired: 7 in]
      n57 = call-poly "Get Config Key.vi"("error in (no error)"=w190, "key"="gradient_calibrations", "section"=w189) -> ("error out"=w179:errorcluster, "value"=w188:string)  [unwired: 7 in]
      n58 = call-poly "Get Config Key.vi"("error in (no error)"=w179, "key"="gradient_supplies", "section"=w170) -> ("error out"=w176:errorcluster, "value"=w178:string)  [unwired: 7 in]
      n59 = call-poly "Get Config Key.vi"("error in (no error)"=w176, "default value"="GPIB0::12::INSTR", "key"="lockin_address", "section"=w170) -> ("error out"=w167:errorcluster, "value"=w173:string)  [unwired: 6 in]
      n60 = call-poly "Get Config Key.vi"("error in (no error)"=w167, "default value"="rri", "key"="magnet_type", "section"=w170) -> ("error out"=w153:errorcluster, "value"=w166:string)  [unwired: 6 in]
      n61 = call-poly "Get Config Key.vi"("error in (no error)"=w153, "default value"=55.0, "key"="sweep_limit", "section"=w115) -> ("error out"=w152:errorcluster, "value"=w150:dbl)  [unwired: 6 in]
      n62 = call-poly "Get Config Key.vi"("error in (no error)"=w152, "default value"=4.0, "key"="mod_limit", "section"=w115) -> ("error out"=w144:errorcluster, "value"=w147:dbl)  [unwired: 6 in]
      n63 = call-poly "Get Config Key.vi"("error in (no error)"=w144, "key"="reverse_sweep_slope", "section"=w115) -> ("error out"=w143:errorcluster, "value"=w142:dbl)  [unwired: 7 in]
      n64 = call-poly "Get Config Key.vi"("error in (no error)"=w143, "key"="reverse_sweep_offset", "section"=w115) -> ("error out"=w139:errorcluster, "value"=w141:dbl)  [unwired: 7 in]
      n65 = call-poly "Get Config Key.vi"("error in (no error)"=w139, "key"="afc_volts_mhz", "section"=w115) -> ("error out"=w122:errorcluster, "value"=w120:dbl)  [unwired: 7 in]
      n66 = call-poly "Get Config Key.vi"("error in (no error)"=w122, "default value"=100.0, "key"="spo2_volts", "section"=w115) -> ("error out"=w116:errorcluster, "value"=w119:dbl)  [unwired: 6 in]
      n67 = call-poly "Get Config Key.vi"("error in (no error)"=w116, "default value"=250.0, "key"="heartrate_volts", "section"=w115) -> ("error out"=w112:errorcluster, "value"=w114:dbl)  [unwired: 6 in]
      n68 = call-poly "Get Config Key.vi"("error in (no error)"=w112, "default value"="Dev1/ai0" ("name to assign"), "key"="thermocouple_channel" ("name to assign"), "section"="hardware" ("name to assign")) -> ("error out"=w111:errorcluster, "value"=w107:string)  [unwired: 6 in]
      n69 = case shown="\"triangle\"" w265 {
        tunnel: [T7."Sine Wave" ("Sweep Waveform") T7."Triangle Wave" ("Sweep Waveform") T7."Sawtooth" ("Sweep Waveform")] -> w263
        frame "sine" {
        }
        frame "triangle" {
        }
        frame "sawtooth", Default {
        }
      }
      n70 = To Lower Case(string=w166) -> (all lower case string=w165:string)
      n71 = Match Pattern(string=w233, regular expression="-") -> (before substring=w235:string)  [unwired: 1 in, 3 out]
      n72 = case shown="\"barda\"" w165 {
        tunnel: [T6."BARDA" ("Magnet Type") T6."Whole Body Permanent" ("Magnet Type") T6."RRI Electromagnet" ("Magnet Type") T6."RRI" ("Magnet Type")] -> w164
        frame "barda" {
        }
        frame "whole_body" {
        }
        frame "rri_electromagnet" {
        }
        frame "rri", Default {
        }
      }
      n73 = Type Cast(type=tag "" ("physical channels"), x=w107) -> (*(type *) &x=w106:tag)
      n74 = Spreadsheet String To Array(delimiter (Tab)=",", format string="%s", spreadsheet string=w125, array type (2D Dbl)=string[][] []) -> (array=w133:string[][])
      n75 = Reverse String(1:w235) -> (0:w236:string)
      n76 = Spreadsheet String To Array(delimiter (Tab)=",", format string="%s", spreadsheet string=w156, array type (2D Dbl)=string[][] []) -> (array=w161:string[][])
      n77 = Spreadsheet String To Array(delimiter (Tab)=",", format string="%s", spreadsheet string=w202, array type (2D Dbl)=string[][] []) -> (array=w206:string[][])
      n78 = Type Cast(type=refnum<visa-resource-name> refnum ("Lock-in Address"), x=w173) -> (*(type *) &x=w171:refnum<visa-resource-name>)
      n79 = To Unsigned Word Integer(number=w288) -> (unsigned 16bit integer=w289:u16)
      n80 = To Unsigned Word Integer(number=w302) -> (unsigned 16bit integer=w303:u16)
      n81 = To Unsigned Word Integer(number=w294) -> (unsigned 16bit integer=w295:u16)
      n82 = Index Array(array=w133, index (row)=0) -> (element=w132:string[])  [unwired: 1 in]
      n83 = Spreadsheet String To Array(delimiter (Tab)=",", format string="%f", spreadsheet string=w188, array type (2D Dbl)=string[][] []) -> (array=w195:string[][])
      n84 = String Subset(string=w236, length (rest)=3 ("length (rest)")) -> (substring=w238:string)  [unwired: 1 in]
      n85 = Spreadsheet String To Array(delimiter (Tab)=",", format string="%s", spreadsheet string=w178, array type (2D Dbl)=string[][] []) -> (array=w185:string[][])
      n86 = Index Array(array=w161, index (row)=0) -> (element=w162:string[])  [unwired: 1 in]
      n87 = Index Array(array=w206, index (row)=0) -> (element=w205:string[])  [unwired: 1 in]
      n88 = for {
        tunnel: w132 -> [w334] mode=indexing
        tunnel: [w330] -> _ mode=indexing
        tunnel: [w328] -> w131 mode=indexing
        tunnel: [w327] -> w130 mode=indexing
        tunnel: [w326] -> w129 mode=indexing
        n89 = call <vilib>:"Trim Whitespace.vi"("string"=w334) -> ("trimmed string"=w333:string)  [unwired: 1 in]
        n90 = To Lower Case(string=w333) -> (all lower case string=w330:string)
        n91 = Equal?(x="x", y=w330) -> (x = y?=w328:bool)
        n92 = Equal?(x="y", y=w330) -> (x = y?=w327:bool)
        n93 = Equal?(x="z", y=w330) -> (x = y?=w326:bool)
      }
      n94 = Reverse String(1:w238) -> (0:w232:string)
      n95 = Fract/Exp String To Number(use system decimal point (T)=FALSE, string=w195) -> (number=w197:dbl[][])  [unwired: 2 in, 1 out]
      n96 = Index Array(array=w185, index (row)=0) -> (element=w186:string[])  [unwired: 1 in]
      n97 = for {
        tunnel: w162 -> [w336] mode=indexing
        tunnel: [w335] -> w155 mode=indexing
        n98 = call <vilib>:"Trim Whitespace.vi"("string"=w336) -> ("trimmed string"=w335:string)  [unwired: 1 in]
      }
      n99 = for {
        tunnel: w205 -> [w344] mode=indexing
        tunnel: [w343] -> w201 mode=indexing
        n100 = call <vilib>:"Trim Whitespace.vi"("string"=w344) -> ("trimmed string"=w343:string)  [unwired: 1 in]
      }
      n101 = Decimal String To Number(string=w232) -> (number=w231:i32)  [unwired: 2 in, 1 out]
      n102 = Index Array(array=w197, index (row)=0) -> (element=w187:dbl[])  [unwired: 1 in]
      n103 = for {
        tunnel: w186 -> [w342] mode=indexing
        tunnel: [w341] -> w175 mode=indexing
        n104 = call <vilib>:"Trim Whitespace.vi"("string"=w342) -> ("trimmed string"=w341:string)  [unwired: 1 in]
      }
      n105 = Or Array Elements(Boolean array=w131) -> (logical OR=w128:bool)
      n106 = Or Array Elements(Boolean array=w130) -> (logical OR=w127:bool)
      n107 = Or Array Elements(Boolean array=w129) -> (logical OR=w126:bool)
      n108 = Build Array(w128, w127, w126) -> (w124:bool[])
      n109 = Bundle By Name(cluster=w325, "Scan Calibration [G/V]"=w321, "Modulation Calibration [G/V]"=w316, "Modulation Phase [deg]"=w313, "Modulation Frequency [Hz]"=w309, "Attenuation [dB]"=w303, "Input Channel Count"=w298, "Time constant"=w295, "Sensitivity"=w289, "Magnet Rotation"=w286, "Balance Scaling Factor"=w280, "Phase Error Scaling Factor"=w276, "AFC Error Scaling Factor"=w272, "Frequency Counter ID"=w269, "Sweep Waveform"=w263, "Q-Factor Scale"=w260, "Q-Data Scale"=w256, "Q-Data Offset"=w253, "Magnet Rotation Slope"=w246, "Magnet Rotation Offset"=w242, "Hardware Version Number"=w233, "Spectrometer ID Number"=w231, "Camera Names"=w155, "Spectrometer Name"=w227, "Lock in Saturation"=w224, "Balance Threshold"=w220, "Phase Error Threshold"=w217, "AFC Error Threshold"=w214, "Linear Actuator Length"=w211, "Gradient Addresses"=w201, "Active Gradients (X Y Z)"=w124, "Gradient Calibrations [G/A*mm]"=w187, "Gradient Power Supplies"=w175, "Lock-in Address"=w171, "Magnet Type"=w164, "Sweep Limit [Gauss]"=w150, "Modulation Limit [Gauss]"=w147, "Reverse Sweep Slope [sec]"=w142, "Reverse Sweep Offset [G]"=w141, "AFC Field Correction [V/MHz]"=w120, "AFC"=TRUE, "SpO2 Calibration [SpO2/V]"=w119, "Heart Rate Calibration [BPM/V]"=w114, "Thermocouple Channel"=w106) -> (w324:T3)
    }
    frame #2 {
      w367 = FALSE ("QA Session?")
      w348 = "reporting" ("section")
      w436 = "web" ("section")
      w421 = "general" ("section")
      w426 = "logging" ("section")
      n110 = call-poly "Get Config Key.vi"("error in (no error)"=w424, "key"="session_number", "section"=w426) -> ("error out"=w428:errorcluster, "value"=w454:i32)  [unwired: 7 in]
      n111 = call-poly "Get Config Key.vi"("error in (no error)"=w428, "key"="safe_shutdown", "section"=w426) -> ("error out"=w427:errorcluster, "value"=w423:bool)  [unwired: 7 in]
      n112 = call-poly "Get Config Key.vi"("error in (no error)"=w427, "default value"=path "C:/Data/EPR Data", "key"="data_path", "section"=w421) -> ("error out"=w422:errorcluster, "value"=w452:path)  [unwired: 6 in]
      n113 = call-poly "Get Config Key.vi"("error in (no error)"=w422, "key"="daq_mode", "section"=w421) -> ("error out"=w420:errorcluster, "value"=w418:string)  [unwired: 7 in]
      n114 = call-poly "Get Config Key.vi"("error in (no error)"=w420, "key"="username", "section"=w436) -> ("error out"=w434:errorcluster, "value"=w451:string)  [unwired: 7 in]
      n115 = call-poly "Get Config Key.vi"("error in (no error)"=w434, "key"="password", "section"=w436) -> ("error out"=w433:errorcluster, "value"=w447:string)  [unwired: 7 in]
      n116 = call-poly "Get Config Key.vi"("error in (no error)"=w433, "key"="login_url", "section"=w436) -> ("error out"=w432:errorcluster, "value"=w446:string)  [unwired: 7 in]
      n117 = call-poly "Get Config Key.vi"("error in (no error)"=w432, "key"="upload_url", "section"=w436) -> ("error out"=w431:errorcluster, "value"=w445:string)  [unwired: 7 in]
      n118 = call-poly "Get Config Key.vi"("error in (no error)"=w431, "key"="success_url", "section"=w436) -> ("error out"=w430:errorcluster, "value"=w442:string)  [unwired: 7 in]
      n119 = call-poly "Get Config Key.vi"("error in (no error)"=w430, "key"="tooth_xml_url", "section"=w436) -> ("error out"=w429:errorcluster, "value"=w440:string)  [unwired: 7 in]
      n120 = call-poly "Get Config Key.vi"("error in (no error)"=w429, "key"="resonator_url", "section"=w436) -> ("error out"=w413:errorcluster, "value"=w438:string)  [unwired: 7 in]
      n121 = call-poly "Get Config Key.vi"("error in (no error)"=w413, "key"="grand_mean", "section"=w348) -> ("error out"=w410:errorcluster, "value"=w411:dbl)  [unwired: 7 in]
      n122 = call-poly "Get Config Key.vi"("error in (no error)"=w410, "key"="slope", "section"=w348) -> ("error out"=w407:errorcluster, "value"=w408:dbl)  [unwired: 7 in]
      n123 = call-poly "Get Config Key.vi"("error in (no error)"=w407, "key"="alpha0", "section"=w348) -> ("error out"=w402:errorcluster, "value"=w404:dbl)  [unwired: 7 in]
      n124 = call-poly "Get Config Key.vi"("error in (no error)"=w402, "key"="alpha1", "section"=w348) -> ("error out"=w395:errorcluster, "value"=w401:dbl)  [unwired: 7 in]
      n125 = call-poly "Get Config Key.vi"("error in (no error)"=w395, "key"="alpha2", "section"=w348) -> ("error out"=w394:errorcluster, "value"=w399:dbl)  [unwired: 7 in]
      n126 = call-poly "Get Config Key.vi"("error in (no error)"=w394, "key"="alpha3", "section"=w348) -> ("error out"=w391:errorcluster, "value"=w397:dbl)  [unwired: 7 in]
      n127 = call-poly "Get Config Key.vi"("error in (no error)"=w391, "key"="alpha4", "section"=w348) -> ("error out"=w390:errorcluster, "value"=w393:dbl)  [unwired: 7 in]
      n128 = call-poly "Get Config Key.vi"("error in (no error)"=w390, "key"="alpha5", "section"=w348) -> ("error out"=w387:errorcluster, "value"=w389:dbl)  [unwired: 7 in]
      n129 = call-poly "Get Config Key.vi"("error in (no error)"=w387, "key"="alpha6", "section"=w348) -> ("error out"=w382:errorcluster, "value"=w386:dbl)  [unwired: 7 in]
      n130 = call-poly "Get Config Key.vi"("error in (no error)"=w382, "key"="dose_correction", "section"=w348) -> ("error out"=w381:errorcluster, "value"=w384:bool)  [unwired: 7 in]
      n131 = call-poly "Get Config Key.vi"("error in (no error)"=w381, "key"="report_dose", "section"=w348) -> ("error out"=w376:errorcluster, "value"=w380:bool)  [unwired: 7 in]
      n132 = call-poly "Get Config Key.vi"("error in (no error)"=w376, "key"="sd_threshold", "section"=w348) -> ("error out"=w375:errorcluster, "value"=w372:dbl)  [unwired: 7 in]
      n133 = call-poly "Get Config Key.vi"("error in (no error)"=w375, "key"="sd_model", "section"=w348) -> ("error out"=w374:errorcluster, "value"=w371:dbl)  [unwired: 7 in]
      n134 = call-poly "Get Config Key.vi"("error in (no error)"=w374, "key"="dosimetric_threshold", "section"=w348) -> ("error out"=w373:errorcluster, "value"=w370:dbl)  [unwired: 7 in]
      n135 = call-poly "Get Config Key.vi"("error in (no error)"=w373, "key"="add_intrasession_errors", "section"=w348) -> ("error out"=w365:errorcluster, "value"=w369:bool)  [unwired: 7 in]
      n136 = call-poly "Get Config Key.vi"("error in (no error)"=w365, "key"="oxy_tolerance_phase", "section"=w348) -> ("error out"=w364:errorcluster, "value"=w359:dbl)  [unwired: 7 in]
      n137 = call-poly "Get Config Key.vi"("error in (no error)"=w364, "key"="oxy_tolerance_center", "section"=w348) -> ("error out"=w363:errorcluster, "value"=w358:dbl)  [unwired: 7 in]
      n138 = call-poly "Get Config Key.vi"("error in (no error)"=w363, "key"="oxy_exclude", "section"=w348) -> ("error out"=w351:errorcluster, "value"=w357:bool)  [unwired: 7 in]
      n139 = call-poly "Get Config Key.vi"("error in (no error)"=w351, "key"="save_ppt", "section"=w348) -> ("error out"=w352:errorcluster, "value"=w349:bool)  [unwired: 7 in]
      n140 = To Lower Case(string=w418) -> (all lower case string=w417:string)
      n141 = Multiply(x=3.141592653589793, y=w359) -> (x*y=w355:dbl)
      n142 = case shown="\"engineering\", Default" w417 {
        tunnel: [enum16{"Engineering", "Dosimetry", "Oximetry"}."Engineering" ("DAQ Mode") enum16{"Engineering", "Dosimetry", "Oximetry"}."Dosimetry" ("DAQ Mode") enum16{"Engineering", "Dosimetry", "Oximetry"}."Oximetry" ("DAQ Mode")] -> w416
        frame "engineering", Default {
        }
        frame "dosimetry" {
        }
        frame "oximetry" {
        }
      }
      n143 = Divide(x=w355, y=180.0) -> (x/y=w353:dbl)
      n144 = Bundle By Name(cluster="Dose Calibration Cluster", "Dose Response.grand_mean"=w411, "Dose Response.slope"=w408, "Dose Correction.a0"=w404, "Dose Correction.a1"=w401, "Dose Correction.a2"=w399, "Dose Correction.a3"=w397, "Dose Correction.a4"=w393, "Dose Correction.a5"=w389, "Dose Correction.a6"=w386, "Dose Correction.Dose Correction"=w384, "Dose Reporting.Reporting is"=w380, "Dose Reporting.sd_threshold [AU]"=w372, "Dose Reporting.sd_model [Gy]"=w371, "Dose Reporting.dosimetric_threshold [Gy]"=w370, "Dose Reporting.Add intrasession errors is"=w369) -> (w414:T1)
      n145 = Bundle By Name(cluster=w456, "Session Number"=w454, "Safe Shutdown?"=w423, "Data file path"=w452, "DAQ Mode"=w416, "Database Username"=w451, "Database Password"=w447, "Database Login URL"=w446, "Database Upload URL"=w445, "Database Success URL"=w442, "Database XML URL"=w440, "Database Resonator URL"=w438, "Dose Calibration Cluster"=w414, "Sample Type"=Sample_Type."Empty Resonator", "QA Session?"=w367, "Report pO2/Scan"=w367, "Temperature [C]"=nan, "Oxy Phase Exclusion Tolerance [rad]"=w353, "Oxy Center Exclusion Tolerance [%]"=w358, "Oxy Exclude Unacceptable"=w357, "Save Session PPT"=w349) -> (w437:T4)
    }
  }
  "Measurement Information Out" <- w8
  "Acquisition Parameters Out" <- w5
  "Hardware Parameters Out" <- w4
  n146 = call "Add Error.vi"("error in (no error)"=w2) -> ("error out"=→"error out":errorcluster)  [unwired: 10 in]
